vi "_GetParameterList.vi"(8 "GUI Method":T1 {"Mass Ranges"."Res" items=["High/High", "Medium/Medium", "Low/Low", "High/Medium", "High/Low", "Medium/High", "Medium/Low", "Low/High", "Low/Medium"]}) -> (0 "DetectorVoltage":string, 1 "Detector":string[][](table)=[["Detector Deflector", "15"], ["Discriminator", "12"], ["Detector Voltage", "2350"], ["Detector Horn", "5500"]], 2 "Source":string[][](table)=[["Drying Gas", "40"], ["Nebulizer Gas 1", "0"], ["Heating Gas 1", "0"], ["Nebulizer Gas 2", "100"], ["Heating Gas 2", "0"], ["Source Exhaust", "0"], ["HSID Temperature", "200"], ["Source 1 Temp", "0"], ["Source 2 Temp", "0"], ["ElectroSpray V1", "3850"], ["ElectroSpray V2", "3850"], ["Curtain Cap", "1000"]], 3 "Instrument":string[][](table)=[["Multipole 1 RF", "350"], ["Entrance Voltage", "35"], ["Entrance Deflector", "0"], ["Multipole 1", "5"], ["Multipole Lens 1", "0"], ["Multipole 2", "0"], ["Multipole Lens 2", "0"], ["Prefilter", "-15"], ["Collision Cell Lens 1", "-10"], ["Collision Cell Lens 2", "-100"], ["Collision Energy", "-50"], ["Axial Field", "100"], ["Collision Cell Lens 3", "-120"], ["Collision Cell Lens 4", "-65"], ["Collision Pressure", "0"]], 4 "Resolution":string[][](table)=[["Quadrupole 1", "15"], ["Quadrupole 2", "3000"]])   [LabVIEW 2015]
uses:
  Type/_GUI Method.ctl
  Type/_Lens Property.ctl
  Type/_Mass Range Property.ctl
  Type/_Mass Range Parameters.ctl
  Type/_RT Res Type.ctl
  Type/_Run Mode.ctl
  Type/_Model Family.ctl
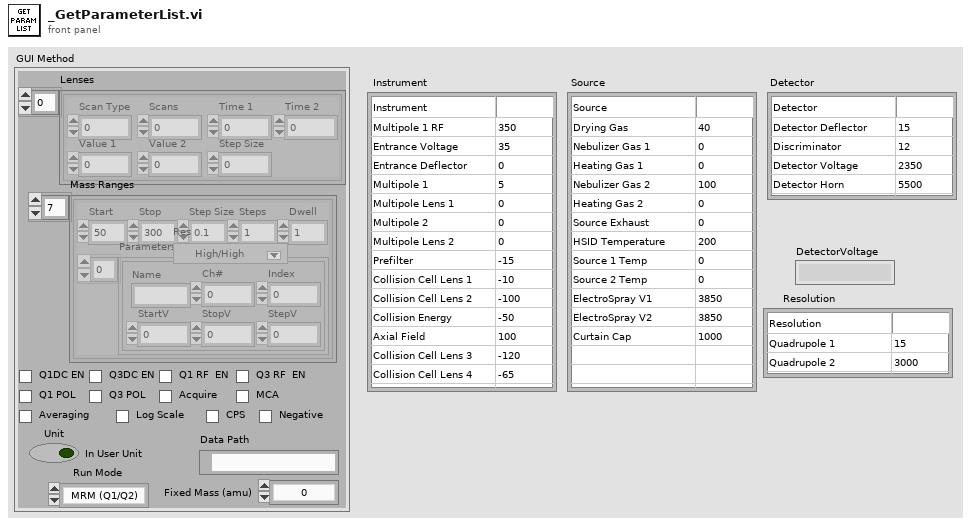
[diagram p1: front panel]
types:
  T1 = typedef "_GUI Method.ctl" = cluster{"Lenses":T2[], "Mass Ranges":T3[], "Acquire":bool, "MCA":bool, "Q1DC EN":bool, "Q1 POL":bool, "Q3 POL":bool, "Q1 RF  EN":bool, "Averaging":bool, "Log Scale":bool, "CPS":bool, "Unit":bool, "Data Path":path, "Run Mode":T6, "Fixed Mass (amu)":dbl, "Q3DC EN":bool, "Q3 RF  EN":bool, "Negative":bool}
  T2 = typedef "_Lens Property.ctl" = cluster{"Scan Type":u8, "Scans":i32, "Time 1":dbl, "Time 2":dbl, "Value 1":dbl, "Value 2":dbl, "Step Size":dbl}
  T3 = typedef "_Mass Range Property.ctl" = cluster{"Start":dbl, "Stop":dbl, "Step Size":dbl, "Steps":i32, "Dwell":dbl, "Parameters":T4[], "Res":T5}
  T4 = typedef "_Mass Range Parameters.ctl" = cluster{"Name":string, "Ch#":u8, "StartV":dbl, "StopV":dbl, "StepV":dbl, "Index":u8}
  T5 = typedef "_RT Res Type.ctl" = u16
  T6 = typedef "_Run Mode.ctl" = enum16{"MRM (Q1/Q2)", "Q1 Scan", "Q1 SRM", "Q2 Scan", "Q2 SRM", "Product Scan", "Precursor Scan", "Neutral Loss", "Neutral Gain"}
  T7 = typedef "_Model Family.ctl" = u16
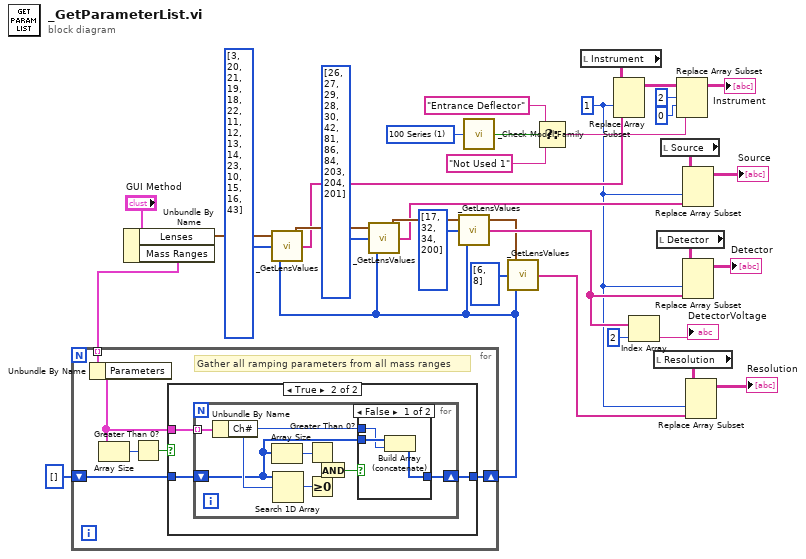
[diagram p0: block diagram]
diagram:
  w22 = T7 1 items=["8080 Series", "100 Series", "200 Series", "300 Series", "Other Series"] ("Model Family (100)")
  w9 = 1 ("disabled index (col)")
  n1 = Unbundle By Name("GUI Method") -> ("Lenses"=w34:T2[], "Mass Ranges"=w3:T3[])
  n2 = for {
    tunnel: w3 -> [w41] mode=indexing
    shift-right: [w39] -> w1
    shift-left: u8[] [] -> [w40]
    # "Gather all ramping parameters from all mass ranges"
    n3 = Unbundle By Name(w41) -> ("Parameters"=w36:T4[])
    n4 = Array Size(array=w36) -> (size(s)=w38:i32)
    n5 = Greater Than 0?(x=w38) -> (x > 0?=w37:bool)
    n6 = case shown="True" w37 {
      tunnel: w40 -> [w42 w45]
      tunnel: [w42 w44] -> w39
      tunnel: w36 -> [_ w43]
      frame False {
        # "No ramping parameter found for this mass range"
      }
      frame True {
        n7 = for {
          shift-right: [w46] -> w44
          shift-left: w45 -> [w47]
          tunnel: w43 -> [w54] mode=indexing
          n8 = Unbundle By Name(w54) -> ("Ch#"=w48:u8)
          n9 = Array Size(array=w47) -> (size(s)=w52:i32)
          n10 = Search 1D Array(1D array=w47, element=w48) -> (index of element=w53:i32)  [unwired: 1 in]
          n11 = Greater Than 0?(x=w52) -> (x > 0?=w50:bool)
          n12 = Greater Or Equal To 0?(x=w53) -> (x >= 0?=w51:bool)
          n13 = And(x=w50, y=w51) -> (x .and. y?=w49:bool)
          n14 = case shown="False" w49 {
            tunnel: w48 -> [w56 _]
            tunnel: w47 -> [w57 w58]
            tunnel: [w55 w58] -> w46
            frame False {
              n15 = Build Array (concatenate)(w57, w56) -> (w55:u8[])
            }
            frame True {
            }
          }
        }
      }
    }
  }
  n16 = call "_GetLensValues.vi"("RampingParams"=w1, "Lens List"=u8[] [3, 20, 21, 19, 18, 22, 11, 12, 13, 14, 23, 10, 15, 16, 43], "Lenses"=w34) -> ("UserValues"=w30:string[], "LensesOut"=w33:T2[])  [unwired: 1 in]
  n17 = call "_GetLensValues.vi"("RampingParams"=w1, "Lens List"=u8[] [26, 27, 29, 28, 30, 42, 81, 86, 84, 203, 204, 201], "Lenses"=w33) -> ("UserValues"=w31:string[], "LensesOut"=w32:T2[])  [unwired: 1 in]
  n18 = call "_GetLensValues.vi"("RampingParams"=w1, "Lens List"=u8[] [17, 32, 34, 200], "Lenses"=w32) -> ("UserValues"=w15:string[], "LensesOut"=w12:T2[])  [unwired: 1 in]
  n19 = call "_Check Model Family.vi"("Model Family (100)"=w22) -> ("Yes"=w21:bool)
  n20 = call "_GetLensValues.vi"("RampingParams"=w1, "Lens List"=u8[] [6, 8], "Lenses"=w12) -> ("UserValues"=w8:string[])  [unwired: 1 in, 1 out]
  n21 = Select(t="Entrance Deflector", s=w21, f="Not Used 1") -> (s? t:f=w18:string)
  n22 = local read "Instrument"() -> (w29:string[][])
  n23 = Replace Array Subset(array=w29, new element=w30, index (col)=w9) -> (w20:string[][])  [unwired: 1 in]
  n24 = Index Array(array=w15, index=2) -> (element=→"DetectorVoltage":string)
  n25 = local read "Resolution"() -> (w11:string[][])
  n26 = local read "Detector"() -> (w26:string[][])
  n27 = local read "Source"() -> (w28:string[][])
  n28 = Replace Array Subset(array=w20, new element=w18, index (row)=2, index (col)=0 ("disabled index (col)")) -> (→"Instrument":string[][])
  n29 = Replace Array Subset(array=w28, new element=w31, index (col)=w9) -> (→"Source":string[][])  [unwired: 1 in]
  n30 = Replace Array Subset(array=w26, new element=w15, index (col)=w9) -> (→"Detector":string[][])  [unwired: 1 in]
  n31 = Replace Array Subset(array=w11, new element=w8, index (col)=w9) -> (→"Resolution":string[][])  [unwired: 1 in]
